vi "JSON Timestamp to ISO8601.vi"(10 "To UTC? (F)":bool, 11 "Local Date Time":timestamp format="%<%Y-%m-%dT%H:%M:%S%6u>T") -> (3 "ISO 8601 Date Time":string)   [LabVIEW 2018, in "labview_json.lvlib"]
uses:
  labview_json.lvlib
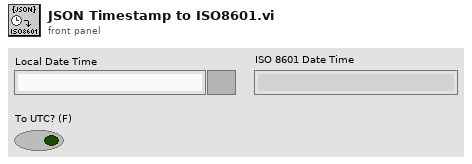
[diagram p1: front panel]
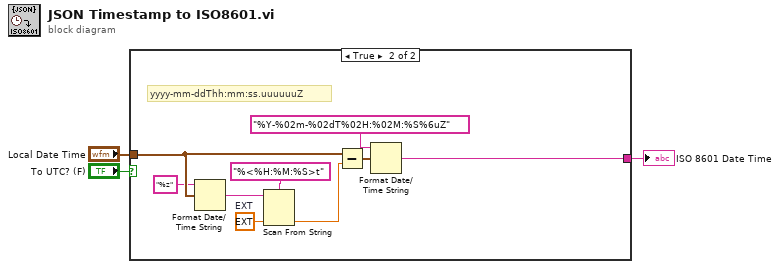
[diagram p0: block diagram]
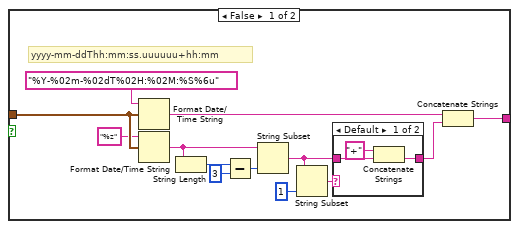
[diagram p2: hidden frame]
diagram:
  n1 = case shown="True" "To UTC? (F)" {
    tunnel: "Local Date Time" -> [w14 w28]
    tunnel: [w12 w26] -> w2
    frame False {
      # "yyyy-mm-ddThh:mm:ss.uuuuuu+hh:mm"
      n2 = Format Date/Time String(time format string (%c)="%Y-%02m-%02dT%02H:%02M:%S%6u", seconds (now)=w14) -> (date/time string=w15:string)  [unwired: 1 in]
      n3 = Format Date/Time String(time format string (%c)="%z", seconds (now)=w14) -> (date/time string=w6:string)  [unwired: 1 in]
      n4 = String Length(string=w6) -> (length=w11:i32)
      n5 = Subtract(x=w11, y=3) -> (x-y=w9:i32)
      n6 = String Subset(string=w6, length (rest)=w9) -> (substring=w4:string)  [unwired: 1 in]
      n7 = String Subset(string=w4, length (rest)=1 ("length (rest)")) -> (substring=w7:string)  [unwired: 1 in]
      n8 = case shown="Default" w7 {
        tunnel: w4 -> [w19 w20]
        tunnel: [w18 w20] -> w5
        frame Default {
          n9 = Concatenate Strings("+" ("string"), w19) -> (w18:string)
        }
        frame "-" {
        }
      }
      n10 = Concatenate Strings(w15, w5) -> (w12:string)
    }
    frame True {
      w23 = ext 0.0  # EXT
      # "yyyy-mm-ddThh:mm:ss.uuuuuuZ"
      n11 = Format Date/Time String(time format string (%c)="%z", seconds (now)=w28) -> (date/time string=w25:string)  [unwired: 1 in]
      n12 = Scan From String(format string="%<%H:%M:%S>t", input string=w25, default 1=w23) -> (output 1=w21:ext)  [unwired: 2 in, 3 out]
      n13 = Subtract(x=w28, y=w21) -> (x-y=w22:timestamp)
      n14 = Format Date/Time String(time format string (%c)="%Y-%02m-%02dT%02H:%02M:%S%6uZ", seconds (now)=w22) -> (date/time string=w26:string)  [unwired: 1 in]
    }
  }
  "ISO 8601 Date Time" <- w2
